vi "CAN Jaguar Get PID.vi"(0 "CAN Jaguar Ref":T1={"Device Number"=0, "Control Mode"=enum."Percent VBus", "Inverted"=FALSE, "Semaphore"=refnum, "Max Vout"=12.0, "DevStatus"={"status"=FALSE, "code"=0, "source"=""}}, 11 "error in (no error)":errorcluster) -> (4 "CAN Jaguar Ref Out":T1={"Device Number"=0, "Control Mode"=enum."Percent VBus", "Inverted"=FALSE, "Semaphore"=refnum, "Max Vout"=12.0, "DevStatus"={"status"=FALSE, "code"=0, "source"=""}}, 6 "P":dbl, 8 "I":dbl, 10 "D":dbl, 15 "error out":errorcluster)   [LabVIEW 2009, in "CAN.lvlib"]
uses:
  CAN.lvlib
  SubVIs/CAN Jaguar Ref.ctl
  SubVIs/CAN Jaguar Control Mode.ctl
  SubVIs/CAN Motor Message IDs.ctl
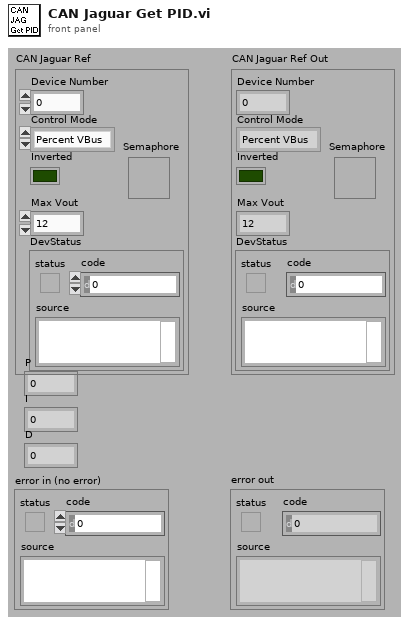
[diagram p1: front panel]
types:
  T1 = typedef "CAN.lvlib/CAN Jaguar Ref.ctl" = cluster{"Device Number":u8, "Control Mode":T2, "Inverted":bool, "Semaphore":T3, "Max Vout":dbl, "DevStatus":errorcluster}
  T2 = typedef "CAN.lvlib/CAN Jaguar Control Mode.ctl" = enum16{"Percent VBus", "Speed", "Position", "Current"}
  T3 = typedef "Semaphore RefNum" = refnum<k1>
  T4 = typedef "CAN.lvlib/CAN Motor Message IDs.ctl" = u32
  T5 = enum16{"big-endian, network order", "native, host order", "little-endian"}
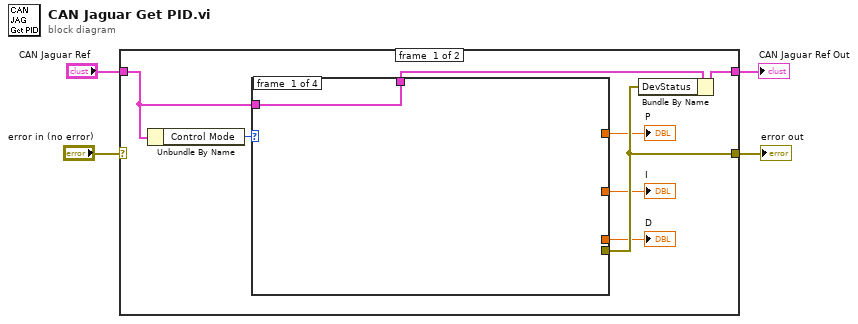
[diagram p0: block diagram]
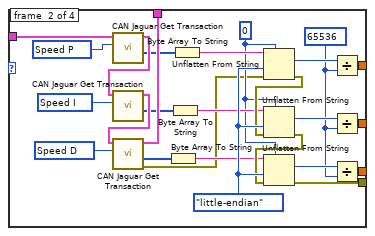
[diagram p2: hidden frame]
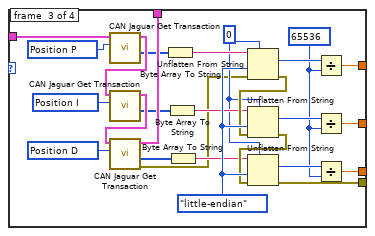
[diagram p3: hidden frame]
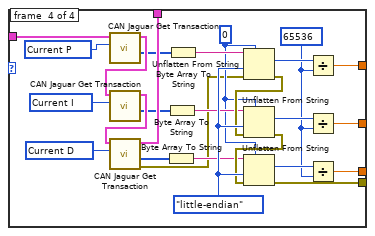
[diagram p4: hidden frame]
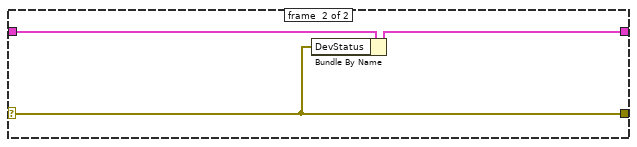
[diagram p5: hidden frame]
diagram:
  n1 = case shown="No Error" "error in (no error)" {
    selector: "error in (no error)" -> [_ w92]
    tunnel: [w12 w93] -> w4
    tunnel: "CAN Jaguar Ref" -> [w6 w94]
    tunnel: [w10 w92] -> w2
    frame #0 {
      n2 = Unbundle By Name(w6) -> ("Control Mode"=w11:T2)
      n3 = case shown="\"Current\"" w11 {
        tunnel: [_ w30 w56 w82] -> w9
        tunnel: [_ w32 w58 w84] -> w10
        tunnel: [_ w28 w54 w80] -> w8
        tunnel: [_ w26 w52 w78] -> w7
        tunnel: w6 -> [w13 w24 w50 w76]
        tunnel: [w13 w18 w44 w69] -> w5
        frame #0 {
        }
        frame #1 {
          w25 = 65536 ("y")
          w22 = T4 33686784 items=["Volt Enable"=33685504, "Volt Disable"=33685568, "Volt Set"=33685632, "Volt Set Ramp"=33685696, "Speed Enable"=33686528, "Speed Disable"=33686592, "Speed Set"=33686656, "Speed P"=33686720, "Speed I"=33686784, "Speed D"=33686848, "Speed Ref"=33686912, "Position Enable"=33688576, "Position Disable"=33688640, "Position Set"=33688704, "Position P"=33688768, "Position I"=33688832, "Position D"=33688896, "Position Ref"=33688960, "Current Enable"=33689600, "Current Disable"=33689664, "Current Set"=33689728, "Current P"=33689792, "Current I"=33689856, "Current D"=33689920, "Status VOut"=33690624, "Status VBus"=33690688, "Status Current"=33690752, "Status Temp"=33690816, "Status Position"=33690880, "Status Speed"=33690944, "Status Limit"=33691008, "Status Fault"=33691072, "Status Power"=33691136, "Config Num Brushes"=33692672, "Config Encoder Lines"=33692736, "Config Pot Turns"=33692800, "Config Brake Coast"=33692864, "Config Limit Mode"=33692928, "Config Limit Fwd"=33692992, "Config Limit Rev"=33693056, "Config Max VOut"=33693120, "Config Fault Time"=33693184, "Motor Ack"=33693696] ("CAN Motor Message IDs")
          w19 = T4 33686848 items=["Volt Enable"=33685504, "Volt Disable"=33685568, "Volt Set"=33685632, "Volt Set Ramp"=33685696, "Speed Enable"=33686528, "Speed Disable"=33686592, "Speed Set"=33686656, "Speed P"=33686720, "Speed I"=33686784, "Speed D"=33686848, "Speed Ref"=33686912, "Position Enable"=33688576, "Position Disable"=33688640, "Position Set"=33688704, "Position P"=33688768, "Position I"=33688832, "Position D"=33688896, "Position Ref"=33688960, "Current Enable"=33689600, "Current Disable"=33689664, "Current Set"=33689728, "Current P"=33689792, "Current I"=33689856, "Current D"=33689920, "Status VOut"=33690624, "Status VBus"=33690688, "Status Current"=33690752, "Status Temp"=33690816, "Status Position"=33690880, "Status Speed"=33690944, "Status Limit"=33691008, "Status Fault"=33691072, "Status Power"=33691136, "Config Num Brushes"=33692672, "Config Encoder Lines"=33692736, "Config Pot Turns"=33692800, "Config Brake Coast"=33692864, "Config Limit Mode"=33692928, "Config Limit Fwd"=33692992, "Config Limit Rev"=33693056, "Config Max VOut"=33693120, "Config Fault Time"=33693184, "Motor Ack"=33693696] ("CAN Motor Message IDs")
          w33 = 0 ("Voltage")
          w23 = T4 33686720 items=["Volt Enable"=33685504, "Volt Disable"=33685568, "Volt Set"=33685632, "Volt Set Ramp"=33685696, "Speed Enable"=33686528, "Speed Disable"=33686592, "Speed Set"=33686656, "Speed P"=33686720, "Speed I"=33686784, "Speed D"=33686848, "Speed Ref"=33686912, "Position Enable"=33688576, "Position Disable"=33688640, "Position Set"=33688704, "Position P"=33688768, "Position I"=33688832, "Position D"=33688896, "Position Ref"=33688960, "Current Enable"=33689600, "Current Disable"=33689664, "Current Set"=33689728, "Current P"=33689792, "Current I"=33689856, "Current D"=33689920, "Status VOut"=33690624, "Status VBus"=33690688, "Status Current"=33690752, "Status Temp"=33690816, "Status Position"=33690880, "Status Speed"=33690944, "Status Limit"=33691008, "Status Fault"=33691072, "Status Power"=33691136, "Config Num Brushes"=33692672, "Config Encoder Lines"=33692736, "Config Pot Turns"=33692800, "Config Brake Coast"=33692864, "Config Limit Mode"=33692928, "Config Limit Fwd"=33692992, "Config Limit Rev"=33693056, "Config Max VOut"=33693120, "Config Fault Time"=33693184, "Motor Ack"=33693696] ("CAN Motor Message IDs")
          w38 = T5."little-endian" ("byte order (0:big-endian, network order)")
          n4 = call "CAN Jaguar Get Transaction.vi"("Message ID"=w23, "CAN Jaguar Ref"=w24) -> ("Data"=w16:u8[], "CAN Jaguar Ref Out"=w21:T1)  [unwired: 1 in, 7 out]
          n5 = call "CAN Jaguar Get Transaction.vi"("Message ID"=w22, "CAN Jaguar Ref"=w21) -> ("Data"=w15:u8[], "CAN Jaguar Ref Out"=w20:T1)  [unwired: 1 in, 7 out]
          n6 = call "CAN Jaguar Get Transaction.vi"("Message ID"=w19, "CAN Jaguar Ref"=w20) -> ("error out"=w17:errorcluster, "Data"=w14:u8[], "CAN Jaguar Ref Out"=w18:T1)  [unwired: 1 in, 6 out]
          n7 = Byte Array To String(unsigned byte array=w14) -> (string=w34:string)
          n8 = Byte Array To String(unsigned byte array=w15) -> (string=w35:string)
          n9 = Byte Array To String(unsigned byte array=w16) -> (string=w39:string)
          n10 = Unflatten From String(type=w33, binary string=w39, byte order (0:big-endian, network order)=w38, error in (no error)=w17) -> (value=w31:i32, error out=w36:errorcluster)  [unwired: 2 out]
          n11 = Unflatten From String(type=w33, binary string=w35, byte order (0:big-endian, network order)=w38, error in (no error)=w36) -> (value=w29:i32, error out=w37:errorcluster)  [unwired: 2 out]
          n12 = Unflatten From String(type=w33, binary string=w34, byte order (0:big-endian, network order)=w38, error in (no error)=w37) -> (value=w27:i32, error out=w32:errorcluster)  [unwired: 2 out]
          n13 = Divide(x=w31, y=w25) -> (x/y=w30:dbl)
          n14 = Divide(x=w29, y=w25) -> (x/y=w28:dbl)
          n15 = Divide(x=w27, y=w25) -> (x/y=w26:dbl)
        }
        frame #2 {
          w51 = 65536 ("y")
          w47 = T4 33688832 items=["Volt Enable"=33685504, "Volt Disable"=33685568, "Volt Set"=33685632, "Volt Set Ramp"=33685696, "Speed Enable"=33686528, "Speed Disable"=33686592, "Speed Set"=33686656, "Speed P"=33686720, "Speed I"=33686784, "Speed D"=33686848, "Speed Ref"=33686912, "Position Enable"=33688576, "Position Disable"=33688640, "Position Set"=33688704, "Position P"=33688768, "Position I"=33688832, "Position D"=33688896, "Position Ref"=33688960, "Current Enable"=33689600, "Current Disable"=33689664, "Current Set"=33689728, "Current P"=33689792, "Current I"=33689856, "Current D"=33689920, "Status VOut"=33690624, "Status VBus"=33690688, "Status Current"=33690752, "Status Temp"=33690816, "Status Position"=33690880, "Status Speed"=33690944, "Status Limit"=33691008, "Status Fault"=33691072, "Status Power"=33691136, "Config Num Brushes"=33692672, "Config Encoder Lines"=33692736, "Config Pot Turns"=33692800, "Config Brake Coast"=33692864, "Config Limit Mode"=33692928, "Config Limit Fwd"=33692992, "Config Limit Rev"=33693056, "Config Max VOut"=33693120, "Config Fault Time"=33693184, "Motor Ack"=33693696] ("CAN Motor Message IDs")
          w48 = T4 33688896 items=["Volt Enable"=33685504, "Volt Disable"=33685568, "Volt Set"=33685632, "Volt Set Ramp"=33685696, "Speed Enable"=33686528, "Speed Disable"=33686592, "Speed Set"=33686656, "Speed P"=33686720, "Speed I"=33686784, "Speed D"=33686848, "Speed Ref"=33686912, "Position Enable"=33688576, "Position Disable"=33688640, "Position Set"=33688704, "Position P"=33688768, "Position I"=33688832, "Position D"=33688896, "Position Ref"=33688960, "Current Enable"=33689600, "Current Disable"=33689664, "Current Set"=33689728, "Current P"=33689792, "Current I"=33689856, "Current D"=33689920, "Status VOut"=33690624, "Status VBus"=33690688, "Status Current"=33690752, "Status Temp"=33690816, "Status Position"=33690880, "Status Speed"=33690944, "Status Limit"=33691008, "Status Fault"=33691072, "Status Power"=33691136, "Config Num Brushes"=33692672, "Config Encoder Lines"=33692736, "Config Pot Turns"=33692800, "Config Brake Coast"=33692864, "Config Limit Mode"=33692928, "Config Limit Fwd"=33692992, "Config Limit Rev"=33693056, "Config Max VOut"=33693120, "Config Fault Time"=33693184, "Motor Ack"=33693696] ("CAN Motor Message IDs")
          w59 = 0 ("Voltage")
          w49 = T4 33688768 items=["Volt Enable"=33685504, "Volt Disable"=33685568, "Volt Set"=33685632, "Volt Set Ramp"=33685696, "Speed Enable"=33686528, "Speed Disable"=33686592, "Speed Set"=33686656, "Speed P"=33686720, "Speed I"=33686784, "Speed D"=33686848, "Speed Ref"=33686912, "Position Enable"=33688576, "Position Disable"=33688640, "Position Set"=33688704, "Position P"=33688768, "Position I"=33688832, "Position D"=33688896, "Position Ref"=33688960, "Current Enable"=33689600, "Current Disable"=33689664, "Current Set"=33689728, "Current P"=33689792, "Current I"=33689856, "Current D"=33689920, "Status VOut"=33690624, "Status VBus"=33690688, "Status Current"=33690752, "Status Temp"=33690816, "Status Position"=33690880, "Status Speed"=33690944, "Status Limit"=33691008, "Status Fault"=33691072, "Status Power"=33691136, "Config Num Brushes"=33692672, "Config Encoder Lines"=33692736, "Config Pot Turns"=33692800, "Config Brake Coast"=33692864, "Config Limit Mode"=33692928, "Config Limit Fwd"=33692992, "Config Limit Rev"=33693056, "Config Max VOut"=33693120, "Config Fault Time"=33693184, "Motor Ack"=33693696] ("CAN Motor Message IDs")
          w64 = T5."little-endian" ("byte order (0:big-endian, network order)")
          n16 = call "CAN Jaguar Get Transaction.vi"("Message ID"=w49, "CAN Jaguar Ref"=w50) -> ("Data"=w40:u8[], "CAN Jaguar Ref Out"=w46:T1)  [unwired: 1 in, 7 out]
          n17 = call "CAN Jaguar Get Transaction.vi"("Message ID"=w47, "CAN Jaguar Ref"=w46) -> ("Data"=w41:u8[], "CAN Jaguar Ref Out"=w45:T1)  [unwired: 1 in, 7 out]
          n18 = call "CAN Jaguar Get Transaction.vi"("Message ID"=w48, "CAN Jaguar Ref"=w45) -> ("error out"=w43:errorcluster, "Data"=w42:u8[], "CAN Jaguar Ref Out"=w44:T1)  [unwired: 1 in, 6 out]
          n19 = Byte Array To String(unsigned byte array=w40) -> (string=w65:string)
          n20 = Byte Array To String(unsigned byte array=w41) -> (string=w61:string)
          n21 = Byte Array To String(unsigned byte array=w42) -> (string=w60:string)
          n22 = Unflatten From String(type=w59, binary string=w65, byte order (0:big-endian, network order)=w64, error in (no error)=w43) -> (value=w57:i32, error out=w62:errorcluster)  [unwired: 2 out]
          n23 = Unflatten From String(type=w59, binary string=w61, byte order (0:big-endian, network order)=w64, error in (no error)=w62) -> (value=w55:i32, error out=w63:errorcluster)  [unwired: 2 out]
          n24 = Unflatten From String(type=w59, binary string=w60, byte order (0:big-endian, network order)=w64, error in (no error)=w63) -> (value=w53:i32, error out=w58:errorcluster)  [unwired: 2 out]
          n25 = Divide(x=w57, y=w51) -> (x/y=w56:dbl)
          n26 = Divide(x=w55, y=w51) -> (x/y=w54:dbl)
          n27 = Divide(x=w53, y=w51) -> (x/y=w52:dbl)
        }
        frame #3 {
          w77 = 65536 ("y")
          w74 = T4 33689856 items=["Volt Enable"=33685504, "Volt Disable"=33685568, "Volt Set"=33685632, "Volt Set Ramp"=33685696, "Speed Enable"=33686528, "Speed Disable"=33686592, "Speed Set"=33686656, "Speed P"=33686720, "Speed I"=33686784, "Speed D"=33686848, "Speed Ref"=33686912, "Position Enable"=33688576, "Position Disable"=33688640, "Position Set"=33688704, "Position P"=33688768, "Position I"=33688832, "Position D"=33688896, "Position Ref"=33688960, "Current Enable"=33689600, "Current Disable"=33689664, "Current Set"=33689728, "Current P"=33689792, "Current I"=33689856, "Current D"=33689920, "Status VOut"=33690624, "Status VBus"=33690688, "Status Current"=33690752, "Status Temp"=33690816, "Status Position"=33690880, "Status Speed"=33690944, "Status Limit"=33691008, "Status Fault"=33691072, "Status Power"=33691136, "Config Num Brushes"=33692672, "Config Encoder Lines"=33692736, "Config Pot Turns"=33692800, "Config Brake Coast"=33692864, "Config Limit Mode"=33692928, "Config Limit Fwd"=33692992, "Config Limit Rev"=33693056, "Config Max VOut"=33693120, "Config Fault Time"=33693184, "Motor Ack"=33693696] ("CAN Motor Message IDs")
          w72 = T4 33689920 items=["Volt Enable"=33685504, "Volt Disable"=33685568, "Volt Set"=33685632, "Volt Set Ramp"=33685696, "Speed Enable"=33686528, "Speed Disable"=33686592, "Speed Set"=33686656, "Speed P"=33686720, "Speed I"=33686784, "Speed D"=33686848, "Speed Ref"=33686912, "Position Enable"=33688576, "Position Disable"=33688640, "Position Set"=33688704, "Position P"=33688768, "Position I"=33688832, "Position D"=33688896, "Position Ref"=33688960, "Current Enable"=33689600, "Current Disable"=33689664, "Current Set"=33689728, "Current P"=33689792, "Current I"=33689856, "Current D"=33689920, "Status VOut"=33690624, "Status VBus"=33690688, "Status Current"=33690752, "Status Temp"=33690816, "Status Position"=33690880, "Status Speed"=33690944, "Status Limit"=33691008, "Status Fault"=33691072, "Status Power"=33691136, "Config Num Brushes"=33692672, "Config Encoder Lines"=33692736, "Config Pot Turns"=33692800, "Config Brake Coast"=33692864, "Config Limit Mode"=33692928, "Config Limit Fwd"=33692992, "Config Limit Rev"=33693056, "Config Max VOut"=33693120, "Config Fault Time"=33693184, "Motor Ack"=33693696] ("CAN Motor Message IDs")
          w85 = 0 ("Voltage")
          w75 = T4 33689792 items=["Volt Enable"=33685504, "Volt Disable"=33685568, "Volt Set"=33685632, "Volt Set Ramp"=33685696, "Speed Enable"=33686528, "Speed Disable"=33686592, "Speed Set"=33686656, "Speed P"=33686720, "Speed I"=33686784, "Speed D"=33686848, "Speed Ref"=33686912, "Position Enable"=33688576, "Position Disable"=33688640, "Position Set"=33688704, "Position P"=33688768, "Position I"=33688832, "Position D"=33688896, "Position Ref"=33688960, "Current Enable"=33689600, "Current Disable"=33689664, "Current Set"=33689728, "Current P"=33689792, "Current I"=33689856, "Current D"=33689920, "Status VOut"=33690624, "Status VBus"=33690688, "Status Current"=33690752, "Status Temp"=33690816, "Status Position"=33690880, "Status Speed"=33690944, "Status Limit"=33691008, "Status Fault"=33691072, "Status Power"=33691136, "Config Num Brushes"=33692672, "Config Encoder Lines"=33692736, "Config Pot Turns"=33692800, "Config Brake Coast"=33692864, "Config Limit Mode"=33692928, "Config Limit Fwd"=33692992, "Config Limit Rev"=33693056, "Config Max VOut"=33693120, "Config Fault Time"=33693184, "Motor Ack"=33693696] ("CAN Motor Message IDs")
          w90 = T5."little-endian" ("byte order (0:big-endian, network order)")
          n28 = call "CAN Jaguar Get Transaction.vi"("Message ID"=w75, "CAN Jaguar Ref"=w76) -> ("Data"=w66:u8[], "CAN Jaguar Ref Out"=w73:T1)  [unwired: 1 in, 7 out]
          n29 = call "CAN Jaguar Get Transaction.vi"("Message ID"=w74, "CAN Jaguar Ref"=w73) -> ("Data"=w67:u8[], "CAN Jaguar Ref Out"=w71:T1)  [unwired: 1 in, 7 out]
          n30 = call "CAN Jaguar Get Transaction.vi"("Message ID"=w72, "CAN Jaguar Ref"=w71) -> ("error out"=w70:errorcluster, "Data"=w68:u8[], "CAN Jaguar Ref Out"=w69:T1)  [unwired: 1 in, 6 out]
          n31 = Byte Array To String(unsigned byte array=w68) -> (string=w86:string)
          n32 = Byte Array To String(unsigned byte array=w67) -> (string=w87:string)
          n33 = Byte Array To String(unsigned byte array=w66) -> (string=w91:string)
          n34 = Unflatten From String(type=w85, binary string=w91, byte order (0:big-endian, network order)=w90, error in (no error)=w70) -> (value=w83:i32, error out=w88:errorcluster)  [unwired: 2 out]
          n35 = Unflatten From String(type=w85, binary string=w87, byte order (0:big-endian, network order)=w90, error in (no error)=w88) -> (value=w81:i32, error out=w89:errorcluster)  [unwired: 2 out]
          n36 = Unflatten From String(type=w85, binary string=w86, byte order (0:big-endian, network order)=w90, error in (no error)=w89) -> (value=w79:i32, error out=w84:errorcluster)  [unwired: 2 out]
          n37 = Divide(x=w83, y=w77) -> (x/y=w82:dbl)
          n38 = Divide(x=w81, y=w77) -> (x/y=w80:dbl)
          n39 = Divide(x=w79, y=w77) -> (x/y=w78:dbl)
        }
      }
      "P" <- w9
      "I" <- w8
      "D" <- w7
      n40 = Bundle By Name(cluster=w5, "DevStatus"=w10) -> (w12:T1)
    }
    frame #1 {
      n41 = Bundle By Name(cluster=w94, "DevStatus"=w92) -> (w93:T1)
    }
  }
  "CAN Jaguar Ref Out" <- w4
  "error out" <- w2
